vi "Main.vi"(8 "error in":errorcluster, 11 "Acquire Data in":refnum<class "Acquire Data.lvclass">) -> (0 "error out":errorcluster, 3 "Acquire Data out":refnum<class "Acquire Data.lvclass">)   [LabVIEW 2018, in "Acquire Data.lvclass"]
doc: "The Queued Message Handler of a Worker."
uses:
  Acquire Data.lvclass
  D:/Program Files (x86)/National Instruments/LabVIEW 2018/vi.lib/addons/_Workers/Library/Classes/Worker/Worker.lvclass
  Initialization Data.ctl
  <vilib>/addons/_Workers/Library/Classes/Message Queue/Message Queue.lvclass
  Acquire Data.lvclass/Acquire Data.ctl
  Status.ctl
  <vilib>/addons/_Workers/Library/Classes/Worker/Worker.lvclass/Worker.ctl
  Aging View/Datas.ctl
  <vilib>/addons/_Workers/Library/Classes/Message/Enqueue Message to Self v2.vi
  <vilib>/addons/_Workers/Library/Classes/Message/Enqueue Message to Queue.vi
  <vilib>/addons/_Workers/Library/Classes/Message/Message.lvclass
  Aging View/Aging View.lvclass
  Save Data/Save Data.lvclass
  <vilib>/addons/_Workers/Library/Classes/Worker/Worker.lvclass
  D:/Program Files (x86)/National Instruments/LabVIEW 2018/vi.lib/addons/_Workers/Library/Classes/Workers Object/Workers Object.lvclass
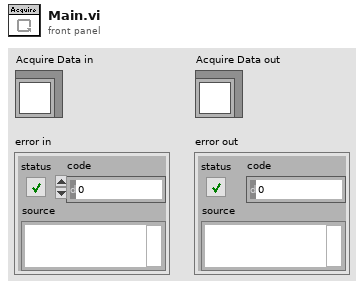
[diagram p1: front panel]
types:
  T1 = typedef "Acquire Data.lvclass/Initialization Data.ctl" = cluster{"AgingView Queue":refnum<class "Message Queue.lvclass">, "SaveData Queue":refnum<class "Message Queue.lvclass">}
  T2 = typedef "Acquire Data.lvclass/Status.ctl" = enum16{"Idle", "Acquire"}
  T3 = typedef "Aging View.lvclass/Datas.ctl" = cluster{"Volts":dbl[], "Currents":dbl[], "Temps":dbl[]}
  T4 = typedef "Workers.lvlib/Case Label.ctl" = string
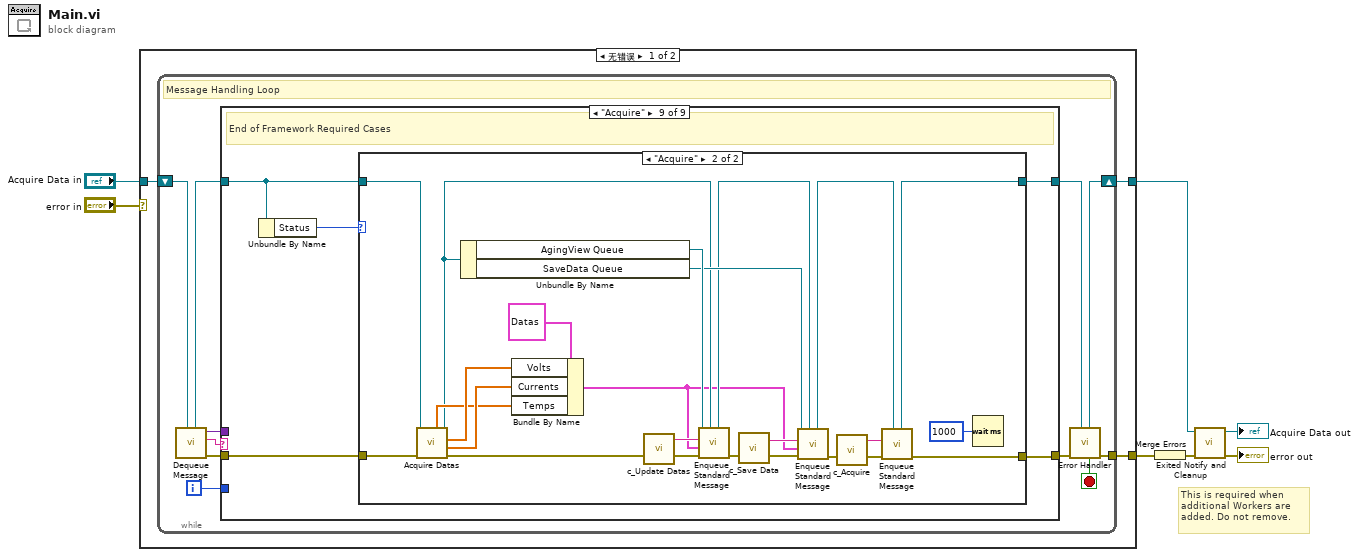
[diagram p0: block diagram]
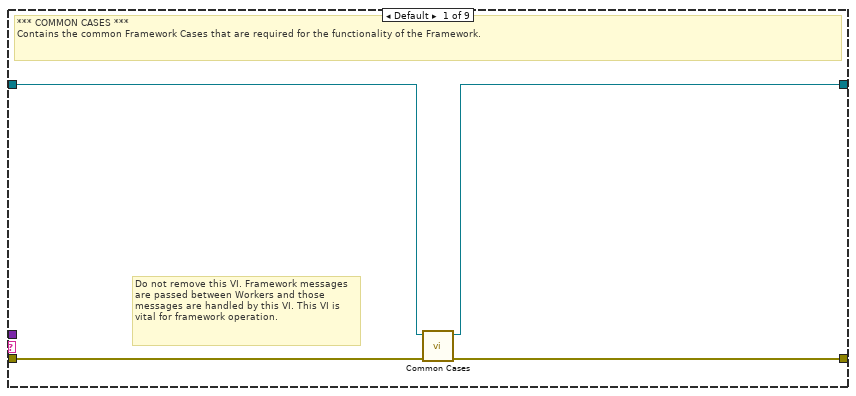
[diagram p2: hidden frame]
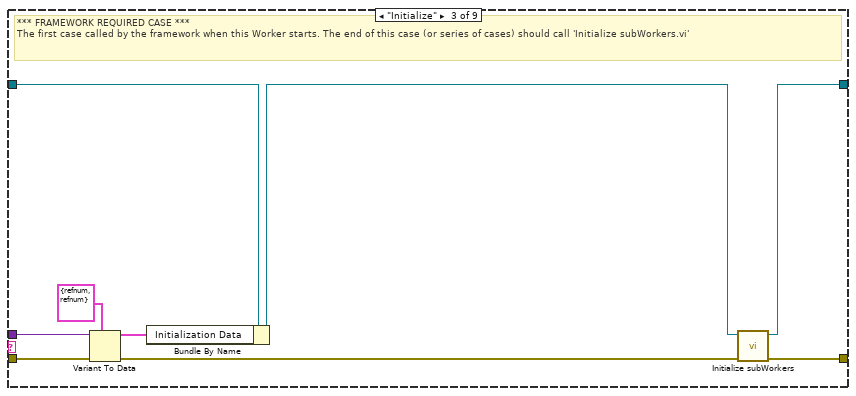
[diagram p4: hidden frame]
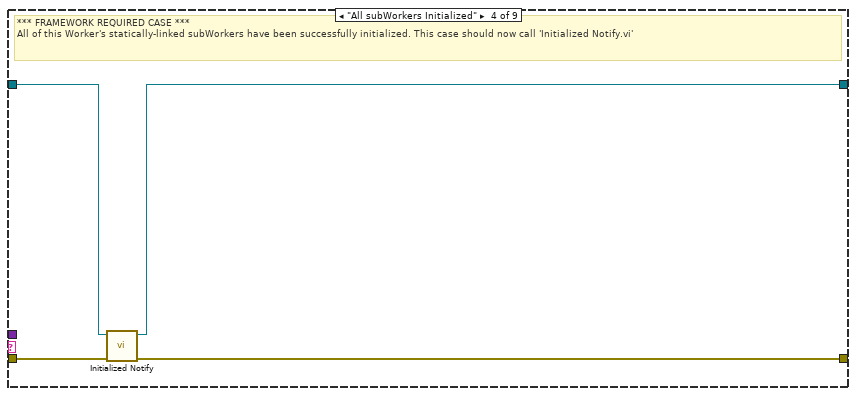
[diagram p5: hidden frame]
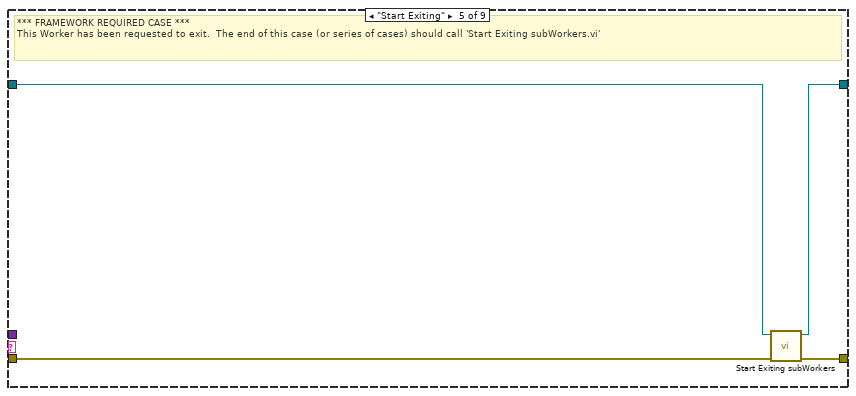
[diagram p6: hidden frame]
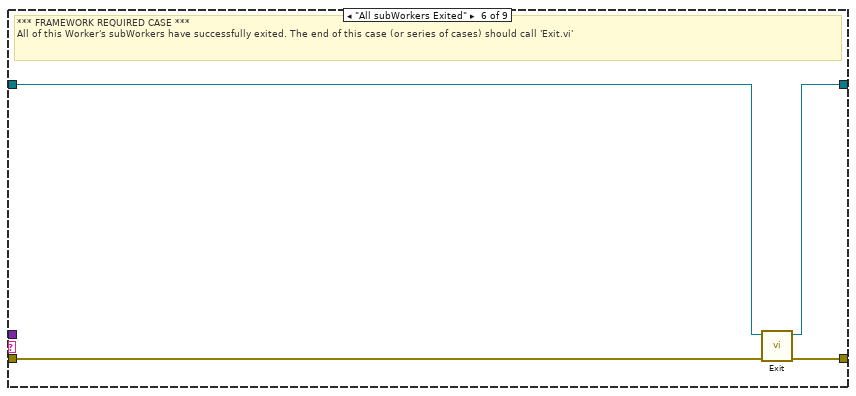
[diagram p7: hidden frame]
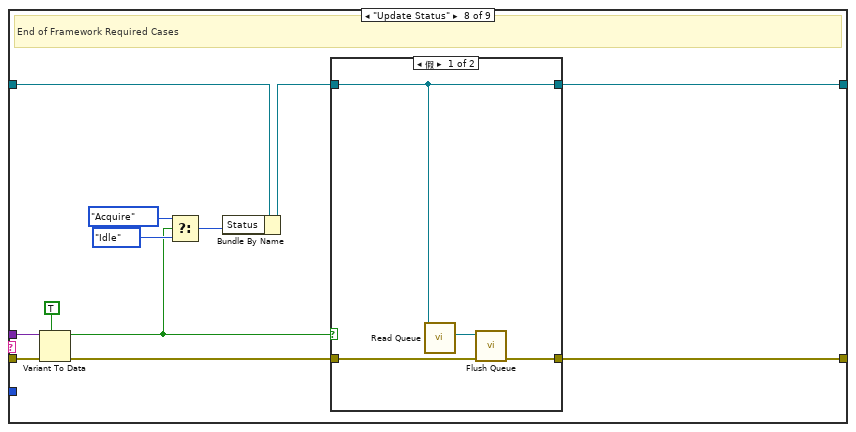
[diagram p9: hidden frame]
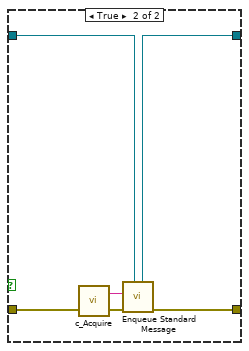
[diagram p10: hidden frame]
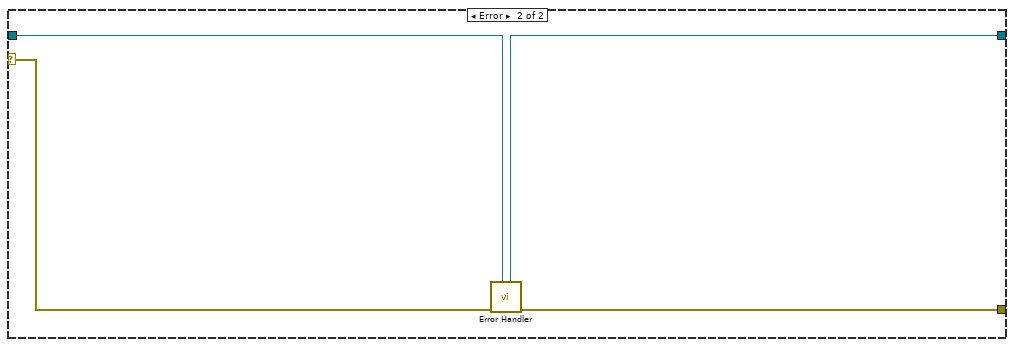
[diagram p12: hidden frame]
diagram:
  # "This is required when additional Workers are added. Do not remove."
  n1 = case shown="无错误" "error in" {
    tunnel: "Acquire Data in" -> [w8 w101]
    tunnel: [w10 w102] -> w6
    tunnel: [w9 w100] -> w7
    selector: "error in" -> [_ w103]
    frame No Error {
      n2 = while {
        shift-right: [w19] -> w9
        shift-left: w8 -> [w21]
        tunnel: [w20] -> w10
        i -> [w11]
        stop <- w12 stop-if-true
        # "Message Handling Loop"
        n3 = call-dynamic "Dequeue Message.vi"("Worker"=w21) -> ("error out"=w18:errorcluster, "Case out"=w13:string, "Data out"=w14:variant, "Worker out"=w16:refnum<class "Acquire Data.lvclass">)  [unwired: 6 in, 1 out]
        n4 = case "Worker MHL Case Structure (DO NOT CHANGE LABEL NAME)" shown="\"Acquire\"" w13 {
          tunnel: w18 -> [w25 w26 w34 w40 w41 w48 w49 w61 w76]
          tunnel: [w24 w26 w36 w39 w44 w47 w49 w53 w74] -> w17
          tunnel: w16 -> [w23 w27 w33 w38 w42 w46 w50 w62 w73]
          tunnel: [w22 w27 w35 w37 w43 w45 w50 w51 w75] -> w15
          tunnel: w14 -> [_ _ w31 _ _ _ _ w60 _]
          tunnel: w11 -> [_ _ _ _ _ _ _ _ _]
          frame Default {
            # "Do not remove this VI. Framework messages are passed between Workers and those messages are handled by this VI. This VI is vital for framework operation."
            # "*** COMMON CASES ***\nContains the common Framework Cases that are required for the functionality of the Framework."
            n5 = call-dynamic "Common Cases.vi"("error in"=w25, "Worker in"=w23) -> ("error out"=w24:errorcluster, "Worker out"=w22:refnum<class "Acquire Data.lvclass">)  [unwired: 8 in]
          }
          frame "------ FRAMEWORK REQUIRED CASES ------" {
            # "Start of Framework Required Cases"
          }
          frame "Initialize" {
            # "*** FRAMEWORK REQUIRED CASE ***\nThe first case called by the framework when this Worker starts. The end of this case (or series of cases) should call 'Initialize subWorkers.vi'"
            n6 = Variant To Data(error in=w34, type=T1 {"AgingView Queue"=refnum, "SaveData Queue"=refnum} ("Cluster"), Variant=w31) -> (data=w28:T1, error out=w32:errorcluster)
            n7 = Bundle By Name(cluster=w33, "Initialization Data"=w28) -> (w30:refnum<class "Acquire Data.lvclass">)
            n8 = call-dynamic "Initialize subWorkers.vi"("error in"=w32, "Worker"=w30) -> ("error out"=w36:errorcluster, "dup Worker out"=w35:refnum<class "Acquire Data.lvclass">)  [unwired: 8 in]
          }
          frame "All subWorkers Initialized" {
            # "*** FRAMEWORK REQUIRED CASE ***\nAll of this Worker's statically-linked subWorkers have been successfully initialized. This case should now call 'Initialized Notify.vi'"
            n9 = call-dynamic "Initialized Notify.vi"("error in"=w40, "Worker"=w38) -> ("error out"=w39:errorcluster, "dup Worker out"=w37:refnum<class "Acquire Data.lvclass">)  [unwired: 8 in]
          }
          frame "Start Exiting" {
            # "*** FRAMEWORK REQUIRED CASE ***\nThis Worker has been requested to exit.  The end of this case (or series of cases) should call 'Start Exiting subWorkers.vi'"
            n10 = call-dynamic "Start Exiting subWorkers.vi"("error_in"=w41, "Worker"=w42) -> ("error out"=w44:errorcluster, "dup Worker out"=w43:refnum<class "Acquire Data.lvclass">)  [unwired: 8 in]
          }
          frame "All subWorkers Exited" {
            # "*** FRAMEWORK REQUIRED CASE ***\nAll of this Worker's subWorkers have successfully exited. The end of this case (or series of cases) should call 'Exit.vi'"
            n11 = call-dynamic "Exit.vi"("error_in"=w48, "Worker"=w46) -> ("error out"=w47:errorcluster, "dup Worker out"=w45:refnum<class "Acquire Data.lvclass">)  [unwired: 8 in]
          }
          frame "-----------------------------------------------" {
            # "End of Framework Required Cases"
          }
          frame "Update Status" {
            # "End of Framework Required Cases"
            n12 = Variant To Data(error in=w61, type=TRUE, Variant=w60) -> (data=w55:bool, error out=w54:errorcluster)
            n13 = Select(t=Status."Acquire" ("Status"), s=w55, f=Status."Idle" ("Status")) -> (s? t:f=w56:T2)
            n14 = Bundle By Name(cluster=w62, "Status"=w56) -> (w52:refnum<class "Acquire Data.lvclass">)
            n15 = case shown="假" w55 {
              tunnel: w54 -> [w66 w71]
              tunnel: [w65 w70] -> w53
              tunnel: w52 -> [w63 w69]
              tunnel: [w63 w68] -> w51
              frame False {
                n16 = call <vilib>:"Read Queue.vi"("Worker"=w63) -> ("Message Queue out"=w64:refnum<class "Message Queue.lvclass">)  [unwired: 9 in, 1 out]
                n17 = call <vilib>:"Flush Queue.vi"("error in (no error)"=w66, "Message Queue"=w64) -> ("error out"=w65:errorcluster)  [unwired: 7 in, 2 out]
              }
              frame True {
                n18 = call "c_Acquire.vi"() -> ("Case Label"=w67:T4)  [unwired: 1 in]
                n19 = call-poly <vilib>:"Enqueue Standard Message.vi"("Worker"=w69, "error in"=w71, "Case Label"=w67) -> ("error out"=w70:errorcluster, "dup Worker out"=w68:refnum<class "Acquire Data.lvclass">)  [unwired: 7 in]
              }
            }
          }
          frame "Acquire" {
            # "End of Framework Required Cases"
            n20 = Unbundle By Name(w73) -> ("Status"=w72:T2)
            n21 = case shown="\"Acquire\"" w72 {
              tunnel: w73 -> [w78 w99]
              tunnel: w76 -> [w77 w98]
              tunnel: [w78 w87] -> w75
              tunnel: [w77 w85] -> w74
              frame "Idle", Default {
              }
              frame "Acquire" {
                n22 = call "Acquire Datas.vi"("error in (no error)"=w98, "Acquire Data in"=w99) -> ("error out"=w94:errorcluster, "Currents"=w96:dbl[], "Volts"=w97:dbl[], "Acquire Data out"=w90:refnum<class "Acquire Data.lvclass">, "Temps"=w95:dbl[])  [unwired: 5 in]
                n23 = Unbundle By Name(w90) -> ("AgingView Queue"=w93:refnum<class "Message Queue.lvclass">, "SaveData Queue"=w91:refnum<class "Message Queue.lvclass">)
                n24 = Bundle By Name(cluster=T3 {"Volts"=[150.16634874669379, 153.68599144269746, 145.2965279660825, 150.72723584964493, 145.24862342605675, 148.81855123547712, 154.16505532014958, 149.4503630674569, 148.93848269644124, 147.4896592075], "Currents"=[150.16634874669379, 153.68599144269746, 145.2965279660825, 150.72723584964493, 145.24862342605675, 148.81855123547712, 154.16505532014958, 149.4503630674569, 148.93848269644124, 147.4896592075], "Temps"=[150.16634874669379, 153.68599144269746, 145.2965279660825, 150.72723584964493, 145.24862342605675, 148.81855123547712, 154.16505532014958, 149.4503630674569, 148.93848269644124, 147.4896592075]} ("Datas"), "Volts"=w97, "Currents"=w96, "Temps"=w95) -> (w79:T3)
                n25 = call "c_Update Datas.vi"() -> ("Case Label"=w84:T4)  [unwired: 1 in]
                n26 = call-poly <vilib>:"Enqueue Standard Message.vi"("Worker"=w90, "error in"=w94, "Data"=w79, "Case Label"=w84, "Message Queue"=w93) -> ("error out"=w92:errorcluster, "dup Worker out"=w89:refnum<class "Acquire Data.lvclass">)  [unwired: 4 in, 1 out]
                n27 = call "c_Save Data.vi"() -> ("Case Label"=w82:T4)  [unwired: 1 in]
                n28 = call-poly <vilib>:"Enqueue Standard Message.vi"("Worker"=w89, "error in"=w92, "Data"=w79, "Case Label"=w82, "Message Queue"=w91) -> ("error out"=w86:errorcluster, "dup Worker out"=w88:refnum<class "Acquire Data.lvclass">)  [unwired: 4 in, 1 out]
                n29 = call "c_Acquire.vi"() -> ("Case Label"=w81:T4)  [unwired: 1 in]
                n30 = call-poly <vilib>:"Enqueue Standard Message.vi"("Worker"=w88, "error in"=w86, "Case Label"=w81) -> ("error out"=w85:errorcluster, "dup Worker out"=w87:refnum<class "Acquire Data.lvclass">)  [unwired: 7 in]
                n31 = Wait (ms)(milliseconds to wait=u32 1000) -> ()  [unwired: 1 out]
              }
            }
          }
        }
        n32 = call-dynamic "Error Handler.vi"("Worker"=w15, "error_in"=w17) -> ("error out"=w20:errorcluster, "Stop Loop"=w12:bool, "Worker out"=w19:refnum<class "Acquire Data.lvclass">)  [unwired: 7 in]
      }
    }
    frame Error {
      n33 = call-dynamic "Error Handler.vi"("Worker"=w101, "error_in"=w103) -> ("error out"=w102:errorcluster, "Worker out"=w100:refnum<class "Acquire Data.lvclass">)  [unwired: 7 in, 1 out]
    }
  }
  n34 = Merge Errors(w6) -> (w3:errorcluster)
  n35 = call-dynamic "Exited Notify and Cleanup.vi"("error_in"=w3, "Worker"=w7) -> ("error out"=→"error out":errorcluster, "dup Worker out"=→"Acquire Data out":refnum<class "Acquire Data.lvclass">)  [unwired: 8 in]
